vi "Sort Spreadsheet by Column.vi"(8 "Error In":errorcluster, 10 "Column Number":i32, 11 "Ref In":refnum<vi>) -> (0 "Error Out":errorcluster)   [LabVIEW 2012]
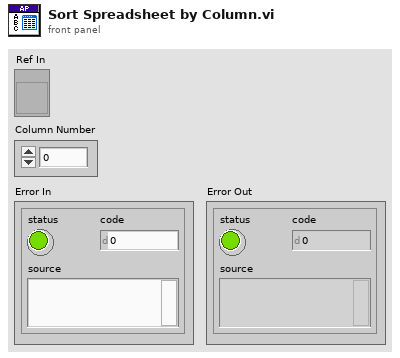
[diagram p1: front panel]
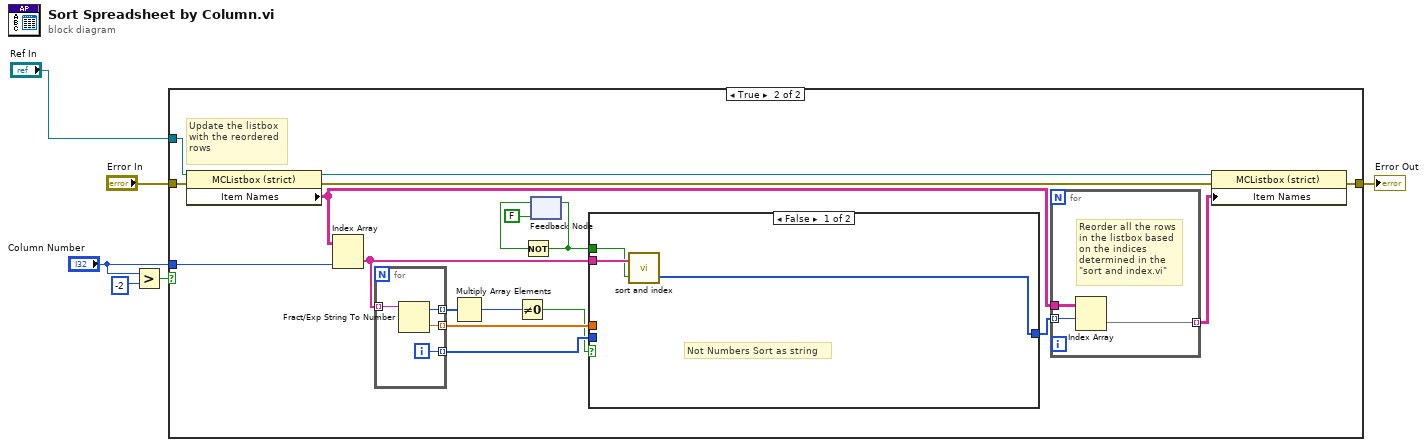
[diagram p0: block diagram]
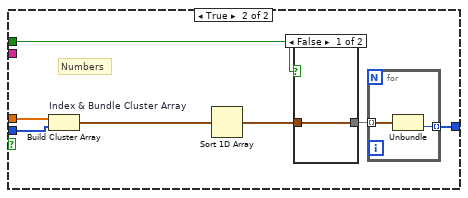
[diagram p3: hidden frame]
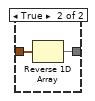
[diagram p4: hidden frame]
diagram:
  n1 = Greater?(x="Column Number", y=-2) -> (0:w6:bool)
  n2 = case shown="True" w6 {
    tunnel: "Column Number" -> [_ w25]
    tunnel: "Ref In" -> [_ w24]
    tunnel: [w7 w19] -> w1
    tunnel: "Error In" -> [w7 w18]
    frame False {
    }
    frame True {
      # "Update the listbox\nwith the reordered\nrows"
      n3 = property class="MCListbox (strict)"(reference=w24, error in=w18) -> (reference out=w20:refnum<vi>, error out=w21:errorcluster, "Item Names"=w23:string[][])
      n4 = Index Array(array=w23, index (col)=w25) -> (element=w10:string[])  [unwired: 1 in]
      n5 = for {
        tunnel: w10 -> [w44] mode=indexing
        tunnel: [w43] -> w13 mode=indexing
        tunnel: [w42] -> w15 mode=indexing
        tunnel: [w41] -> w12 mode=indexing
        i -> [w41]
        n6 = Fract/Exp String To Number(string=w44) -> (offset past number=w42:i32, number=w43:dbl)  [unwired: 3 in]
      }
      n7 = Multiply Array Elements(1:w15) -> (0:w14:i32)
      n8 = Not Equal To 0?(x=w14) -> (x != 0?=w11:bool)
      n9 = feedback #1(FALSE) -> (w17:bool)
      n10 = Not(x=w17) -> (.not. x?=w9:bool)
      n11 = feedback-in #1(w9) -> ()
      n12 = case shown="False" w11 {
        tunnel: w13 -> [_ w35]
        tunnel: w12 -> [_ w34]
        tunnel: [w26 w32] -> w8
        tunnel: w10 -> [w28 _]
        tunnel: w9 -> [w27 w31]
        frame False {
          # "Not Numbers Sort as string"
          n13 = call "sort and index.vi"("Reverse"=w27, "Array to Sort"=w28) -> ("Sorted Indices Array"=w26:i32[])  [unwired: 1 out]
        }
        frame True {
          # "Numbers"
          n14 = Build Cluster Array "Index & Bundle Cluster Array"(w35, w34) -> (w33:cluster{dbl, i32}[])
          n15 = Sort 1D Array(array=w33) -> (sorted array=w30:cluster{dbl, i32}[])
          n16 = case shown="False" w31 {
            tunnel: w30 -> [w36 w38]
            tunnel: [w36 w37] -> w29
            frame False {
            }
            frame True {
              n17 = Reverse 1D Array(array=w38) -> (reversed array=w37:cluster{dbl, i32}[])
            }
          }
          n18 = for {
            tunnel: w29 -> [w40] mode=indexing
            tunnel: [w39] -> w32 mode=indexing
            n19 = Unbundle(w40) -> (w39:i32)  [unwired: 1 out]
          }
        }
      }
      n20 = for {
        tunnel: w8 -> [w46] mode=indexing
        tunnel: w23 -> [w47]
        tunnel: [w45] -> w22 mode=indexing
        # "Reorder all the rows\nin the listbox based\non the indices determined in the \"sort and index.vi\""
        n21 = Index Array(array=w47, index (row)=w46) -> (element=w45:string[])  [unwired: 1 in]
      }
      n22 = property class="MCListbox (strict)"(reference=w20, error in=w21, "Item Names"=w22) -> (error out=w19:errorcluster)  [unwired: 1 out]
    }
  }
  "Error Out" <- w1
